vi "DVR Unflatten.vi"(8 "error in (no error)":errorcluster, 11 "Flatten Data in":u8[](array[numeric])) -> (0 "error out":errorcluster, 2 "DVRs Out":refnum<data-value>[](array[refnum]), 3 "Flatten Data out":u8[](array[numeric]), 5 "Header out":T1)   [LabVIEW 2021, in "CIF_NIChn_FIFO_DAQ_DVR.lvclass"]
uses:
  CIF_NIChn_FIFO_DAQ_DVR.lvclass
  ChannelCommon/typedef/FIFO Header.ctl
  ChannelCommon/typedef/Datatype Waveform.ctl
  ChannelCommon/typedef/Errors.ctl
  <vilib>/CIF Foundation/CIF Utilities/DataTypes/Unflatten I64.vi
  <vilib>/CIF Foundation/CIF Utilities/Errors/Append Error Location.vi
  CIF_NIChn_FIFO_DAQ_DVR.lvclass/CIF_NIChn_FIFO_DAQ_DVR.ctl
  ChannelCommon/ChannelCommon.lvlib
  <vilib>/CIF Foundation/CIF Utilities/DataTypes/DataTypes_CIF_U.lvlib
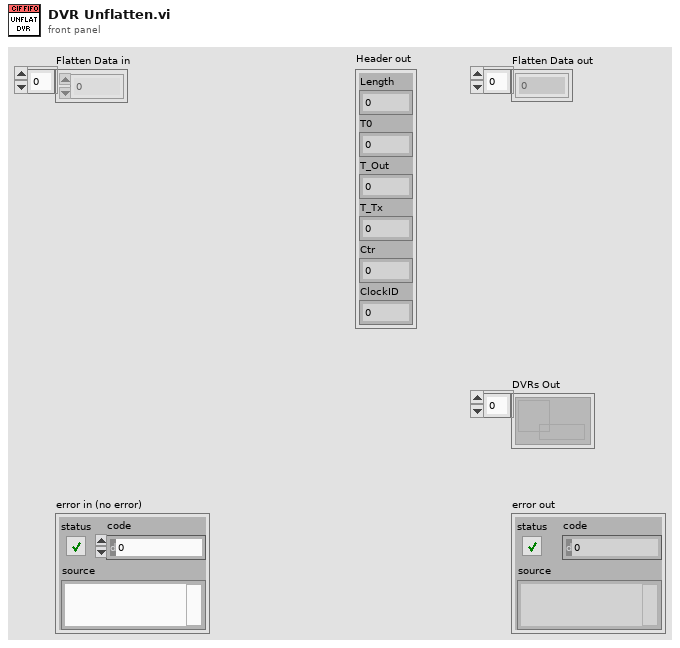
[diagram p1: front panel]
types:
  T1 = typedef "ChannelCommon.lvlib/FIFO Header.ctl" = cluster{"Length":u64, "T0":i64, "T_Out":i64, "T_Tx":i64, "Ctr":u64, "ClockID":u8}
  T2 = typedef "ChannelCommon.lvlib/Errors.ctl" = enum16{"gRPC Server Not Found", "Duplicate Channel", "Missing Channel", "Incorrect Type", "Flatten Error", "Unflatten Data", "Channel Length", "Plugin Connection", "gRPC Server Connection", "FIFO Unflatten", "Required Override", "Remove Not Found"}
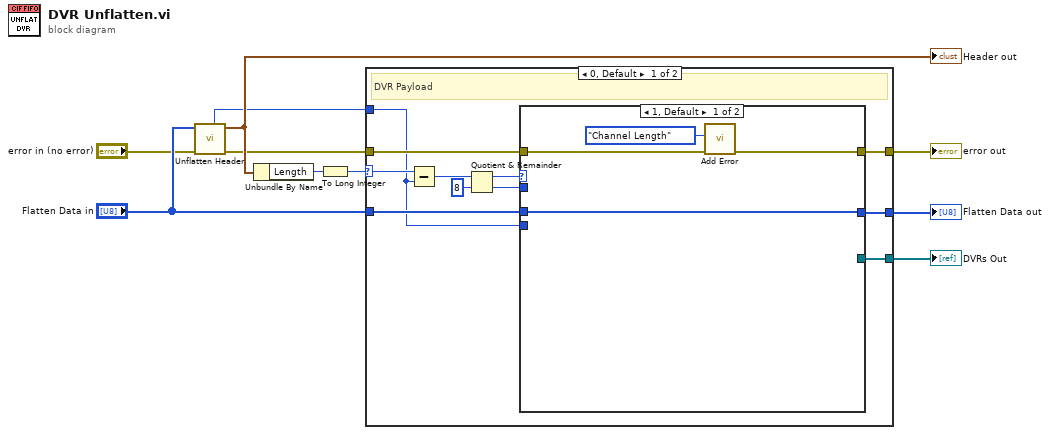
[diagram p0: block diagram]
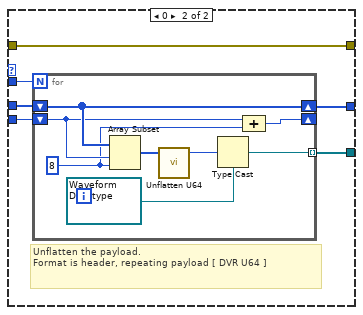
[diagram p2: hidden frame]
diagram:
  n1 = call "Unflatten Header.vi"("error in (no error)"="error in (no error)", "Flattened Data in"="Flatten Data in") -> ("error out"=w2:errorcluster, "Header out"=w7:T1, "offset out"=w1:i32)  [unwired: 7 in]
  "Header out" <- w7
  n2 = Unbundle By Name(w7) -> ("Length"=w8:u64)
  n3 = To Long Integer(number=w8) -> (32bit integer=w6:i32)
  n4 = case shown="0, Default" w6 {
    selector: w6 -> [w17 _]
    tunnel: [w11 _] -> w5
    tunnel: [w21 w40] -> w10
    tunnel: [w20 w41] -> w9
    tunnel: "Flatten Data in" -> [w19 w41]
    tunnel: w2 -> [w18 w40]
    tunnel: w1 -> [w12 _]
    frame 0, Default {
      # "DVR Payload"
      n5 = Subtract(x=w17, y=w12) -> (x-y=w16:i32)
      n6 = Quotient & Remainder(x=w16, y=8) -> (x-y*floor(x/y)=w13:i32, floor(x/y)=w14:i32)
      n7 = case shown="1, Default" w13 {
        tunnel: [_ w26] -> w11
        tunnel: [w23 w27] -> w21
        tunnel: [w25 w31] -> w20
        tunnel: w19 -> [w25 w30]
        tunnel: w18 -> [w24 w27]
        tunnel: w12 -> [_ w29]
        tunnel: w14 -> [_ w28]
        frame 1, Default {
          n8 = call "Add Error.vi"("error in (no error)"=w24, "Error"=Errors."Channel Length") -> ("error out"=w23:errorcluster)  [unwired: 9 in]
        }
        frame 0 {
          # "Unflatten the payload.\nFormat is header, repeating payload [ DVR U64 ]"
          n9 = for {
            N: w28 -> [_]
            shift-right: [w39] -> w31
            shift-left: w30 -> [w39]
            shift-right: [w37] -> _
            shift-left: w29 -> [w38]
            tunnel: [w32] -> w26 mode=indexing
            w36 = 8 ("y")
            n10 = Array Subset(array=w39, index=w38, length=w36) -> (w35:u8[])
            n11 = call <vilib>:"Unflatten U64.vi"("Flat Data"=w35) -> ("U64"=w34:u64)  [unwired: 4 in]
            n12 = Type Cast(type=refnum<data-value> refnum ("element"), x=w34) -> (*(type *) &x=w32:refnum<data-value>)
            n13 = Compound Arithmetic op=ADD(w38, w36) -> (w37:i32)
          }
        }
      }
    }
    frame 48 {
      # "Header only"
    }
  }
  "error out" <- w10
  "Flatten Data out" <- w9
  "DVRs Out" <- w5
